vi "Can_Add.vi"(8 "error in (no error)":errorcluster, 11 "IB_Tree_Item_Proj_MyComputer in":refnum<class "IB_Tree_Item_Proj_MyComputer.lvclass">) -> (0 "error out":errorcluster, 2 "can add?":bool, 3 "IB_Tree_Item_Proj_MyComputer out":refnum<class "IB_Tree_Item_Proj_MyComputer.lvclass">)   [LabVIEW 2020, in "IB_Tree_Item_Proj_MyComputer.lvclass"]
uses:
  <vilib>/AppBuilder/IB_Classes/Tree_Item_Proj_MyComputer/IB_Tree_Item_Proj_MyComputer.lvclass
  <vilib>/AppBuilder/IB_Classes/Tree_Item_Proj_MyComputer/IB_Tree_Item_Proj_MyComputer.lvclass/IB_Tree_Item_Proj_MyComputer.ctl
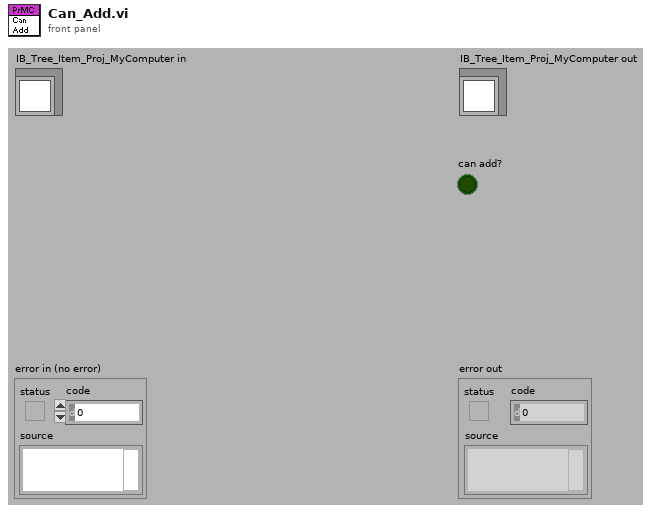
[diagram p1: front panel]
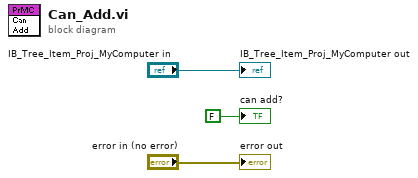
[diagram p0: block diagram]
diagram:
  "error out" <- "error in (no error)"
  "IB_Tree_Item_Proj_MyComputer out" <- "IB_Tree_Item_Proj_MyComputer in"
  "can add?" <- FALSE ("can add?")
